vi "Activity_2(P1).vi"() -> ()   [LabVIEW 2019]
panel:
  out "Temperature Out":string
  out "Temperature In":string
  out "Too Cold":bool
  out "Too Hot":bool
  in  "*F to *C\n\n\n*C to *F":bool
  out "Temperature Out":dbl(slide) scale=-100.0..300.0
  in  "Temperature In":dbl(slide) scale=-100.0..300.0
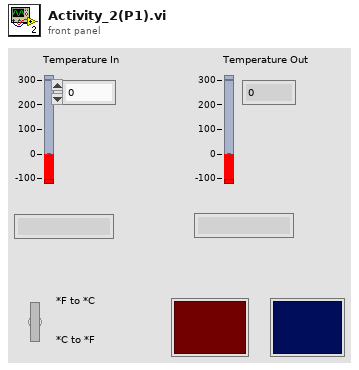
[diagram p1: front panel]
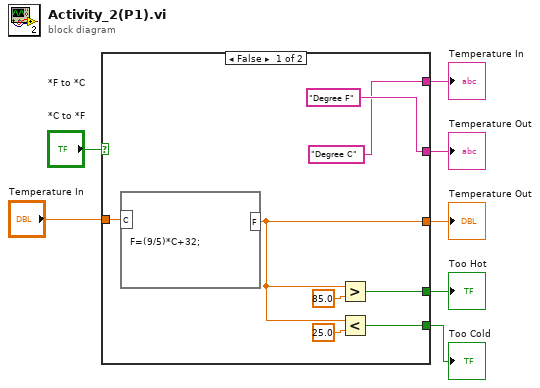
[diagram p0: block diagram]
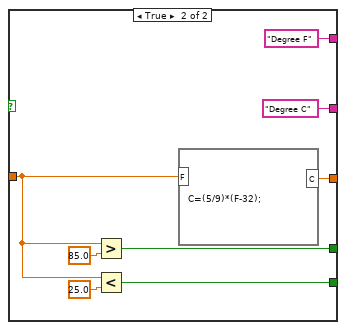
[diagram p2: hidden frame]
diagram:
  n1 = case shown="False" "*F to *C\n\n\n*C to *F" {
    tunnel: "Temperature In" -> [w13 w16]
    tunnel: [w10 w21] -> w5
    tunnel: ["Degree C" "Degree F"] -> w2
    tunnel: ["Degree F" "Degree C"] -> w1
    tunnel: [w12 w18] -> w4
    tunnel: [w11 w17] -> w3
    frame False {
      n2 = formula code="F=(9/5)*C+32;"("C"=w13) -> ("F"=w10:dbl)
      n3 = Greater?(x=w10, y=85.0) -> (0:w12:bool)
      n4 = Less?(x=w10, y=25.0) -> (x < y?=w11:bool)
    }
    frame True {
      n5 = Greater?(x=w16, y=85.0) -> (0:w18:bool)
      n6 = Less?(x=w16, y=25.0) -> (x < y?=w17:bool)
      n7 = formula code="C=(5/9)*(F-32);"("F"=w16) -> ("C"=w21:dbl)
    }
  }
  "Temperature Out" <- w5
  "Too Hot" <- w4
  "Too Cold" <- w3
  "Temperature In" <- w2
  "Temperature Out" <- w1
